vi "Config User Timestamps FIFO.vi"(8 "error in (no error)":errorcluster, 10 "Buffer Size (elements)":u32=10485760, 11 "FPGA Ref in":refnum<k20>) -> (0 "error out":errorcluster, 3 "FPGA Ref out":refnum<k20>)   [LabVIEW 2025]
uses:
  <vilib>/rvi/interface/nirviMethod/nirviMethod.xnode
  <vilib>/FPGAPlugInAG/Dynamic/niLvFpga_ConfigureFifo_Dynamic.vi
  <vilib>/rvi/errors/niLvFpgaMergeErrorWithErrorCode.vi
  <vilib>/FPGAPlugInAG/Dynamic/niLvFpga_StartFifo_Dynamic.vi
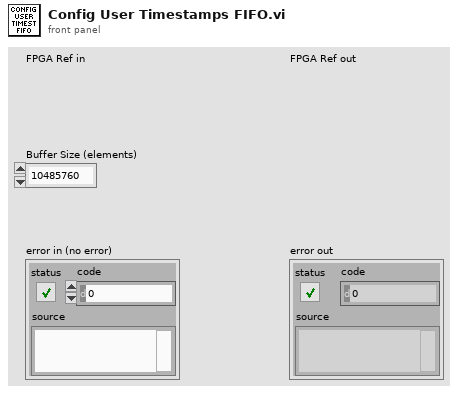
[diagram p1: front panel]
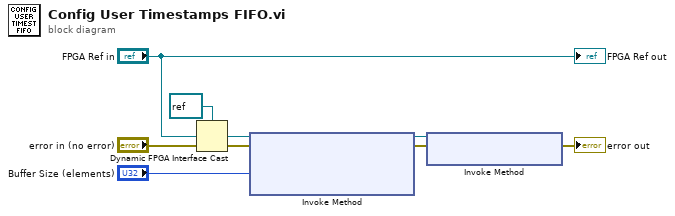
[diagram p0: block diagram]
diagram:
  n1 = Dynamic FPGA Interface Cast(Session In=refnum<k20> refnum ("FPGA VI Reference Out"), Type="FPGA Ref in") -> (Session Out=w3:refnum<k20>)
  n2 = xnode "Invoke Method"("FPGA VI Reference In"=w3, "error in"="error in (no error)", "Requested Depth"="Buffer Size (elements)") -> ("FPGA VI Reference Out"=w4:refnum<k20>, "error out"=w6:errorcluster)  [unwired: 1 out]
  n3 = xnode "Invoke Method"("FPGA VI Reference In"=w4, "error in"=w6) -> ("error out"=→"error out":errorcluster)  [unwired: 1 out]
  "FPGA Ref out" <- "FPGA Ref in"
